vi "FTW-Project-ConditionalDisableSymbols-Get.vi"(0 "Project Ref (blank for Active Project)":refnum<vi>, 5 "Target (Root or My Computer)":string(combo)="Root", 11 "error in":errorcluster) -> (4 "Project out":refnum<vi>, 6 "TargetItem out":refnum<vi>, 8 "Conditional Disable Symbols":variant, 15 "error out":errorcluster)   [LabVIEW 2014]
uses:
  Core/Error/FTW-ERR-ThrowError.vi
panel:
  # "Inputs"
  # "Outputs"
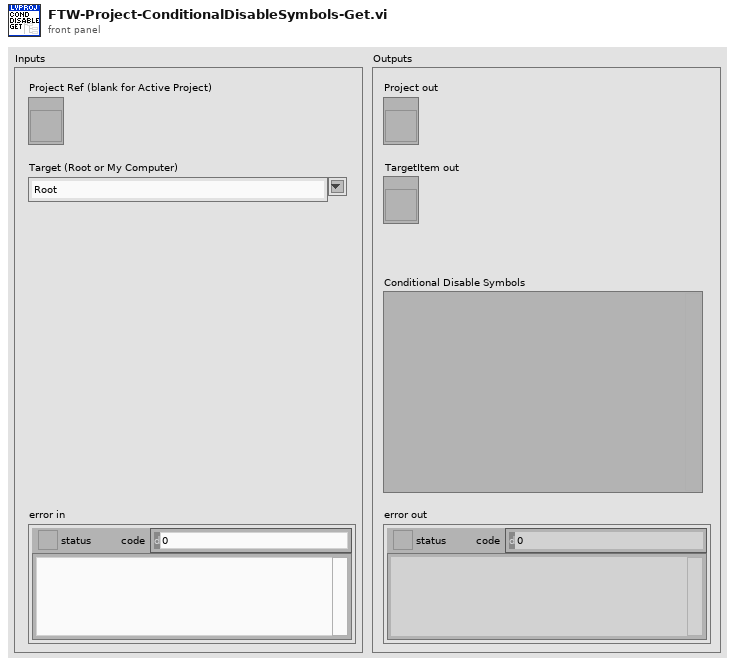
[diagram p1: front panel]
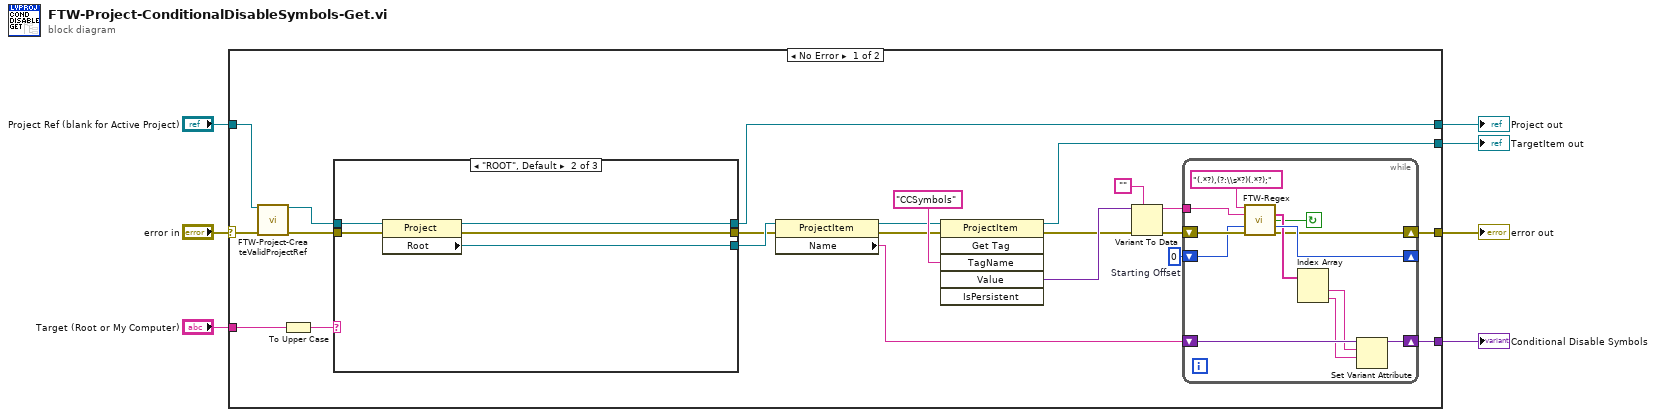
[diagram p0: block diagram]
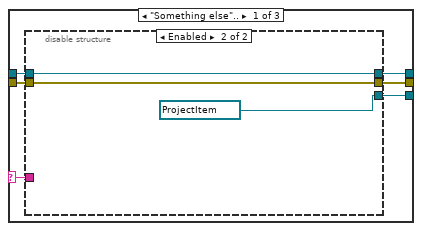
[diagram p2: hidden frame]
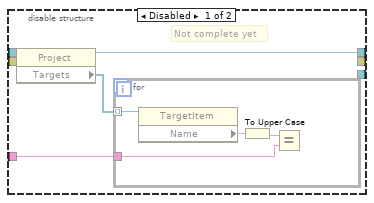
[diagram p3: hidden frame]
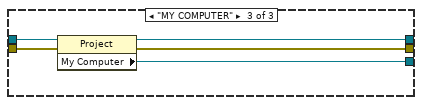
[diagram p4: hidden frame]
diagram:
  n1 = case shown="No Error" "error in" {
    selector: "error in" -> [w26 w71]
    tunnel: [w12 w71] -> w7
    tunnel: "Target (Root or My Computer)" -> [w23 _]
    tunnel: "Project Ref (blank for Active Project)" -> [w27 w70]
    tunnel: [w21 w70] -> w3
    tunnel: [w11 _] -> w2
    tunnel: [w9 _] -> w1
    frame No Error {
      w14 = 0  # Starting Offset
      n2 = call "FTW-Project-CreateValidProjectRef.vi"("Project Ref (blank for Active Project)"=w27, "error in"=w26) -> ("Project Ref"=w25:refnum<vi>, "error out"=w24:errorcluster)  [unwired: 11 in, 1 out]
      n3 = To Upper Case(1:w23) -> (0:w22:string)
      n4 = case shown="\"ROOT\", Default" w22 {
        selector: w22 -> [w45 _ _]
        tunnel: w25 -> [w46 w64 w69]
        tunnel: w24 -> [w47 w63 w68]
        tunnel: [w44 w62 w66] -> w21
        tunnel: [w42 w61 w65] -> w18
        tunnel: [w43 w60 w67] -> w17
        frame "Something else".. {
          n5 = disable-structure shown="Enabled" {
            disable-tunnel: w47 -> [w52 w58]
            disable-tunnel: w46 -> [w51 w59]
            disable-tunnel: w45 -> [w49 _]
            disable-tunnel: [w48 w59] -> w44
            disable-tunnel: [_ w58] -> w43
            disable-tunnel: [_ refnum<vi> refnum ("Root")] -> w42
            frame Disabled {
              # "Not complete yet"
              n6 = property class="Project"(reference=w51, error in=w52) -> (reference out=w48:refnum<vi>, "Targets"=w50:refnum<vi>[])  [unwired: 1 out]
              n7 = for {
                tunnel: w50 -> [w56] mode=indexing
                tunnel: w49 -> [w53]
                n8 = property class="TargetItem"(reference=w56) -> ("Name"=w55:string)  [unwired: 1 in, 2 out]
                n9 = To Upper Case(1:w55) -> (0:w54:string)
                n10 = Equal?(x=w54, y=w53) -> ()  [unwired: 1 out]
              }
            }
            frame Enabled {
            }
          }
        }
        frame "ROOT", Default {
          n11 = property class="Project"(reference=w64, error in=w63) -> (reference out=w62:refnum<vi>, error out=w60:errorcluster, "Root"=w61:refnum<vi>)
        }
        frame "MY COMPUTER" {
          n12 = property class="Project"(reference=w69, error in=w68) -> (reference out=w66:refnum<vi>, error out=w67:errorcluster, "My Computer"=w65:refnum<vi>)
        }
      }
      n13 = property class="ProjectItem"(reference=w18, error in=w17) -> (reference out=w19:refnum<vi>, error out=w16:errorcluster, "Name"=w10:string)
      n14 = invoke class="ProjectItem" method="Get Tag"(reference=w19, error in=w16, "TagName"="CCSymbols" ("Tag Name")) -> (reference out=w9:refnum<vi>, error out=w8:errorcluster, "Value"=w28:variant)  [unwired: 3 in, 3 out]
      n15 = Variant To Data(error in=w8, type="", Variant=w28) -> (data=w13:string, error out=w15:errorcluster)
      n16 = while {
        shift-right: [w39] -> _
        shift-left: w14 -> [w40]
        tunnel: w13 -> [w38]
        shift-right: [w35] -> w12
        shift-left: w15 -> [w41]
        shift-right: [w33] -> w11
        shift-left: w10 -> [w34]
        stop <- w36 continue-if-true
        n17 = call "FTW-Regex.vi"("Regular Expression"="(.*?),(?:\\s*?)(.*?);", "Input String"=w38, "Starting Offset"=w40, "error in"=w41) -> ("Submatches"=w37:string[], "Match Found?"=w36:bool, "Offset after Match"=w39:i32, "error out"=w35:errorcluster)  [unwired: 7 in, 1 out]
        n18 = Index Array(array=w37) -> (element #1=w32:string, element #2=w31:string)  [unwired: 2 in]
        n19 = Set Variant Attribute(Variant=w34, name=w32, value=w31) -> (Variant out=w33:variant)  [unwired: 1 in, 2 out]
      }
    }
    frame Error {
    }
  }
  "error out" <- w7
  "Project out" <- w3
  "Conditional Disable Symbols" <- w2
  "TargetItem out" <- w1
